vi "get_scale.vi"(5 "Field_Astrom":T1 {"CRVAL" format="%.6g"; "CD" format="%_7g"}) -> (0 "teta (deg)":dbl, 1 "Scale (\"/px)":dbl, 2 "Scale (deg/px)":dbl)   [LabVIEW 2010]
uses:
  <vilib>/Analysis/Matrix/Numeric/Conversions/Array To Matrix - RA2.vi
  <vilib>/Analysis/baseanly.llb/Real Determinant.vi
  <vilib>/Analysis/Matrix/NI_Matrix.lvlib
  <vilib>/Analysis/NI_AALBase.lvlib
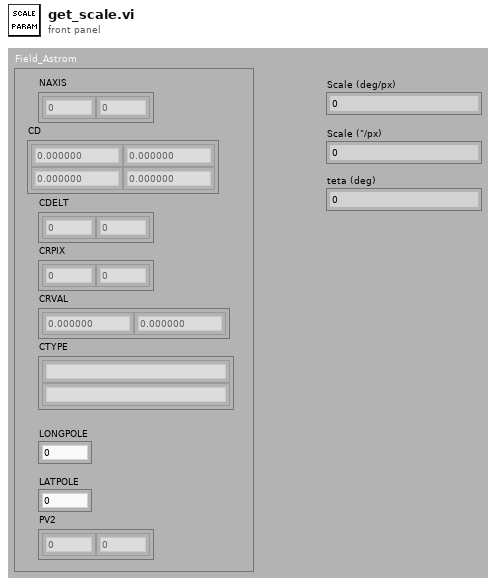
[diagram p1: front panel]
types:
  T1 = cluster{"NAXIS":dbl[], "CD":dbl[][], "CDELT":dbl[], "CRPIX":dbl[], "CTYPE":string[], "CRVAL":dbl[], "LONGPOLE":dbl, "LATPOLE":dbl, "PV2":dbl[]}
  T2 = typedef "NI_Matrix.lvlib/RealMatrix.ctl" = dbl[][]
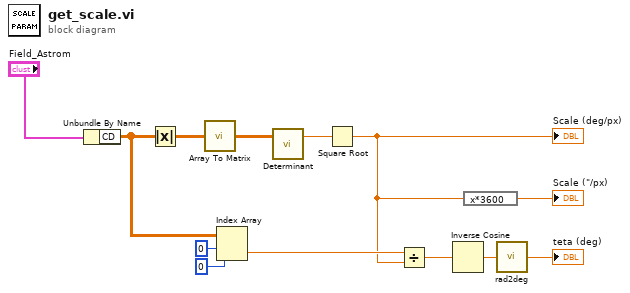
[diagram p0: block diagram]
diagram:
  n1 = Unbundle By Name("Field_Astrom") -> ("CD"=w8:dbl[][])
  n2 = Absolute Value(x=w8) -> (abs(x)=w12:dbl[][])
  n3 = call-poly <vilib>:"Array To Matrix.vi"("Real 2D Array"=w12) -> ("Real Matrix"=w11:T2)
  n4 = Index Array(array=w8, index (row)=0, index (col)=0 ("disabled index (col)")) -> (element=w5:dbl)
  n5 = call-poly <vilib>:"Determinant.vi"("Input Matrix"=w11) -> ("determinant"=w10:dbl)  [unwired: 1 in, 1 out]
  n6 = Square Root(x=w10) -> (sqrt(x)=w4:dbl)
  "Scale (deg/px)" <- w4
  n7 = Divide(x=w5, y=w4) -> (x/y=w3:dbl)
  n8 = Inverse Cosine(1:w3) -> (0:w2:dbl)
  n9 = expression code="x*3600"(w4) -> (→"Scale (\"/px)":dbl)
  n10 = call "rad2deg.vi"("rad"=w2) -> ("deg"=→"teta (deg)":dbl)
